vi "test_thorcam_NET.vi"() -> ()   [LabVIEW 2025]
uses:
  C:/Program Files/Thorlabs/Scientific Imaging/Scientific Camera Support/Scientific Camera Interfaces/LabVIEW/64_bit/Library_X64/Thorlabs.TSI.TLCameraInterfaces.dll
  Program Files/Thorlabs/Scientific Imaging/Scientific Camera Support/Scientific Camera Interfaces/LabVIEW/64_bit/Library_X64/Thorlabs.TSI.TLCameraInterfaces.dll
  C:/Program Files/Thorlabs/Scientific Imaging/Scientific Camera Support/Scientific Camera Interfaces/LabVIEW/64_bit/Library_X64/Thorlabs.TSI.TLCamera.dll
  Program Files/Thorlabs/Scientific Imaging/Scientific Camera Support/Scientific Camera Interfaces/LabVIEW/64_bit/Library_X64/Thorlabs.TSI.TLCamera.dll
  Windows/System32/pvcam64.dll
panel:
  out "error out 4":errorcluster
  out "error out 3":errorcluster
  out "error out 2":errorcluster
  out "arg1":i32
  out "TLCameraSDK reference out":refnum<k24>
  out "error out":errorcluster
  out "Serial Numbers":string[](array[string])
  out "Number of Cameras":i32
  in  "error in (no error)":errorcluster
  out "DiscoverAvailableCameras":refnum<k24>
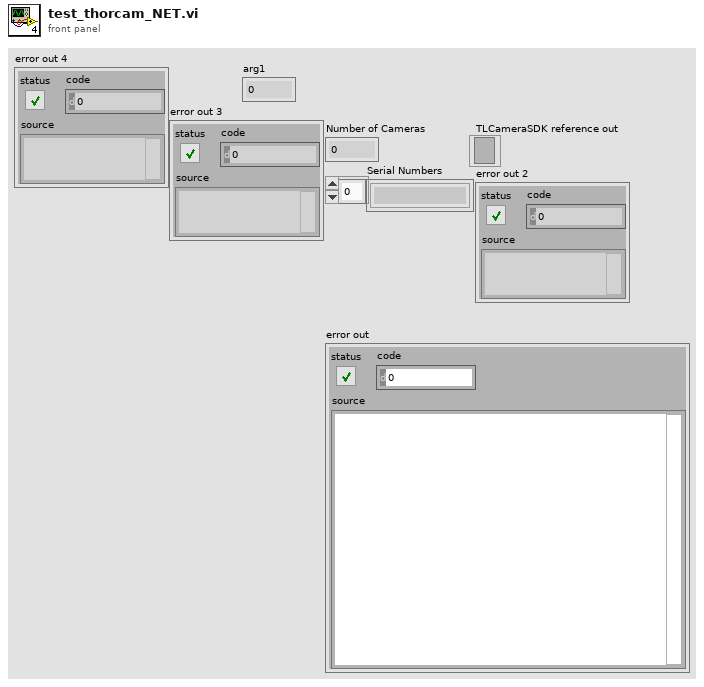
[diagram p1: front panel]
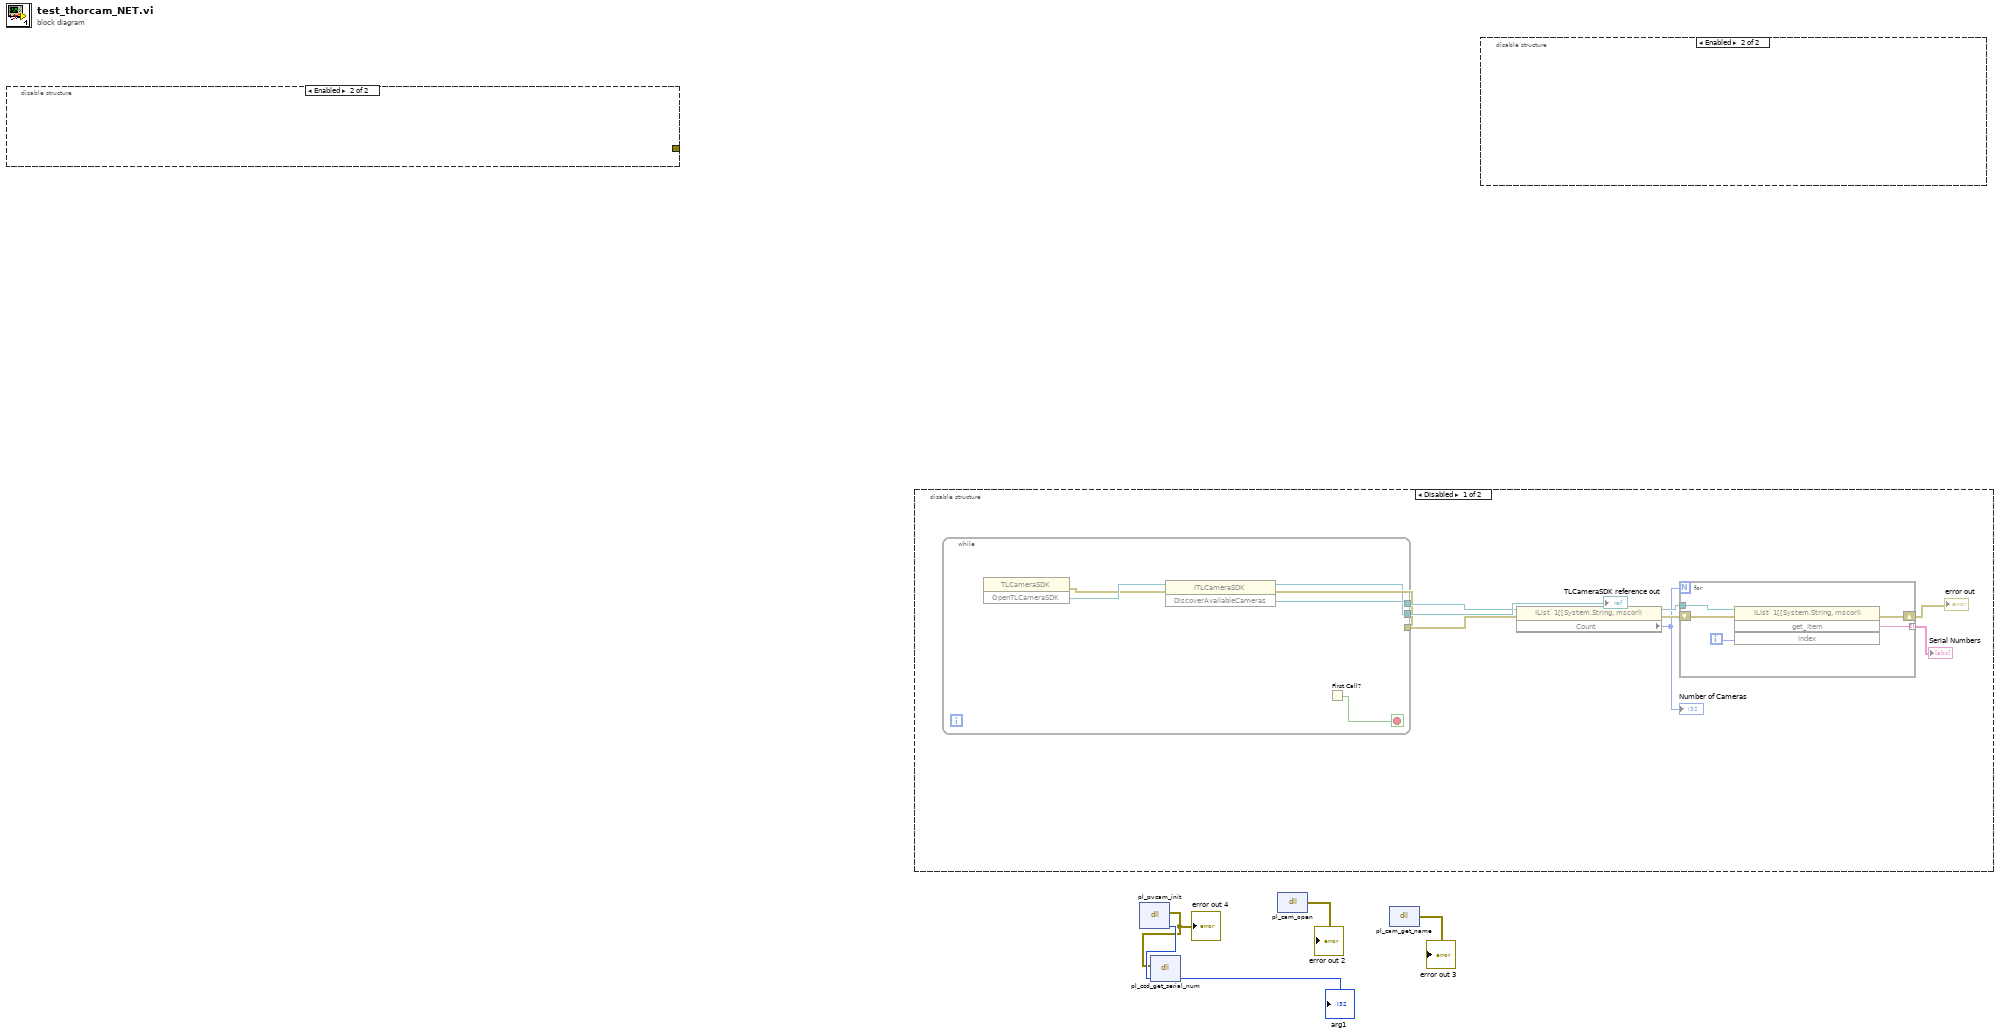
[diagram p0: block diagram]
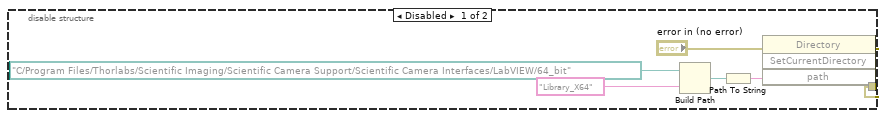
[diagram p3: hidden frame]
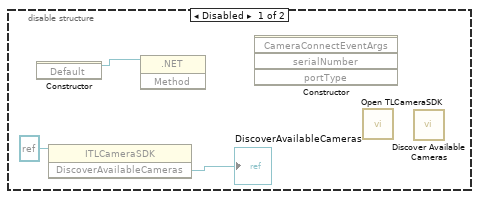
[diagram p4: hidden frame]
diagram:
  n1 = disable-structure shown="Enabled" {
    disable-tunnel: [w6 _] -> _
    frame Disabled {
      n2 = Build Path(base path=path "C:/Program Files/Thorlabs/Scientific Imaging/Scientific Camera Support/Scientific Camera Interfaces/LabVIEW/64_bit", name or relative path="Library_X64") -> (appended path=w9:path)
      n3 = Path To String(path=w9) -> (string=w10:string)
      n4 = invoke class="Directory" method="SetCurrentDirectory"(error in="error in (no error)", "path"=w10) -> (error out=w6:errorcluster)  [unwired: 2 in, 3 out]
    }
    frame Enabled {
    }
  }
  n5 = disable-structure shown="Disabled" {
    frame Disabled {
      n6 = while {
        tunnel: [w28] -> w12
        tunnel: [w27] -> w13
        tunnel: [w26] -> w14
        stop <- w25 stop-if-true
        n7 = invoke class="TLCameraSDK" method="OpenTLCameraSDK"() -> (error out=w29:errorcluster, "OpenTLCameraSDK"=w30:refnum<k24>)  [unwired: 3 in, 1 out]
        n8 = invoke class="ITLCameraSDK" method="DiscoverAvailableCameras"(reference=w30, error in=w29) -> (reference out=w26:refnum<k24>, error out=w28:errorcluster, "DiscoverAvailableCameras"=w27:refnum<k24>)  [unwired: 1 in]
        n9 = First Call?() -> (First Call?: T/F=w25:bool)
      }
      "TLCameraSDK reference out" <- w14
      n10 = property class="IList`1[[System.String, mscorli"(reference=w13, error in=w12) -> (reference out=w16:refnum<k24>, error out=w17:errorcluster, "Count"=w15:i32)
      "Number of Cameras" <- w15
      n11 = for {
        N: w15 -> [_]
        tunnel: w16 -> [w24]
        shift-right: [w22] -> w19
        shift-left: w17 -> [w23]
        tunnel: [w20] -> w18 mode=indexing
        i -> [w21]
        n12 = invoke class="IList`1[[System.String, mscorli" method="get_Item"(reference=w24, error in=w23, "index"=w21) -> (error out=w22:errorcluster, "get_Item"=w20:string)  [unwired: 1 in, 2 out]
      }
      "Serial Numbers" <- w18
      "error out" <- w19
    }
    frame Enabled {
    }
  }
  n13 = dll-call lib="C:/Windows/System32/pvcam64.dll" fn="pl_pvcam_init"() -> (error out=w3:errorcluster, "arg"=w5:i32)  [unwired: 5 in, 1 out]
  "error out 4" <- w3
  n14 = dll-call lib="C:/Windows/System32/pvcam64.dll" fn="pl_ccd_get_serial_num"(error in=w3, "arg1"=w5) -> ("arg1"=→"arg1":i32)  [unwired: 3 in, 2 out]
  n15 = dll-call lib="C:/Windows/System32/pvcam64.dll" fn="pl_cam_open"() -> (error out=→"error out 2":errorcluster)  [unwired: 4 in, 1 out]
  n16 = dll-call lib="C:/Windows/System32/pvcam64.dll" fn="pl_cam_get_name"() -> (error out=→"error out 3":errorcluster)  [unwired: 4 in, 1 out]
  n17 = disable-structure shown="Enabled" {
    frame Disabled {
      n18 = constructor class=".NET"() -> (reference out=w33:refnum<k24>)  [unwired: 3 in, 2 out]
      n19 = invoke class="ITLCameraSDK" method="DiscoverAvailableCameras"(reference=refnum<k24> refnum) -> ("DiscoverAvailableCameras"=→"DiscoverAvailableCameras":refnum<k24>)  [unwired: 2 in, 2 out]
      n20 = invoke class=".NET" method=#-1(reference=w33) -> ()  [unwired: 2 in, 3 out]
      n21 = constructor() -> ()  [unwired: 5 in, 5 out]
      n22 = call "Open TLCameraSDK.vi"() -> ()  [unwired: 10 in, 2 out]
      n23 = call "Discover Available Cameras.vi"() -> ()  [unwired: 8 in, 4 out]
    }
    frame Enabled {
    }
  }
